vi "mlink_ao_scan_wait_until_done.vi"(8 "error in (no error)":errorcluster, 10 "timeout":i32, 11 "connection ID":i32=-1) -> (0 "error out":errorcluster, 3 "connection ID out":i32)   [LabVIEW 2009, in "MicroDAQ.lvlib" / "mlink.lvlib"]
doc: "This function waits for analog output signal generation to complete. The timeout argument specifies the maximum amount of time in milliseconds to wait for the generation to complete. This function returns an error if the time elapses. If timeout is set to -1, the function waits \nindefinitely. it the timeout is set to 0, the function checks once and returns an error if the \nmeasurement or generation is not done"
uses:
  <instrlib>/MicroDAQ/Mlink library wraper/mlink.lvlib
  <instrlib>/MicroDAQ/MLink32.dll
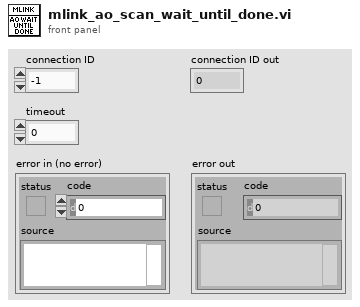
[diagram p1: front panel]
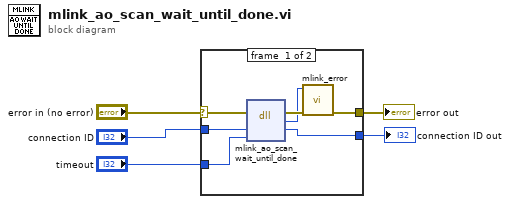
[diagram p0: block diagram]
diagram:
  n1 = case shown="No Error" "error in (no error)" {
    selector: "error in (no error)" -> [w12 w14]
    tunnel: "connection ID" -> [w11 w13]
    tunnel: [w10 w13] -> w3
    tunnel: [w7 w14] -> w2
    tunnel: "timeout" -> [w6 _]
    frame #0 {
      n2 = dll-call lib="C:/Program Files (x86)/National Instruments/LabVIEW 2009/instr.lib/MicroDAQ/MLink32.dll" fn="mlink_ao_scan_wait_until_done" ("MLink64.dll:mlink_dsp_run")(error in=w12, "link_fd"=w11, "timeout"=w6) -> (error out=w9:errorcluster, "return type"=w8:i32, "link_fd"=w10:i32)  [unwired: 3 in, 1 out]
      n3 = call <instrlib>:"mlink_error.vi"("error in (no error)"=w9, "error code"=w8) -> ("error out"=w7:errorcluster)  [unwired: 9 in]
    }
    frame #1 {
    }
  }
  "connection ID out" <- w3
  "error out" <- w2
